vi "DAQ_Initialize.vi"(8 "error in":errorcluster, 11 "ai0 = Temperature\nai1 = Current\nai2 = Torque\nai3 = Vibration\nai4 = RPM":tag) -> (0 "error out":errorcluster, 3 "task out":refnum<k21>)   [LabVIEW 2026]
uses:
  <vilib>/DAQmx/create/channels.llb/DAQmx Create Channel (AI-Voltage-Basic).vi
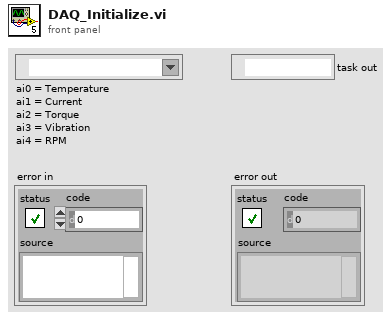
[diagram p1: front panel]
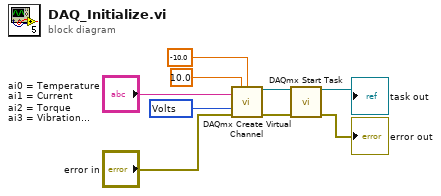
[diagram p0: block diagram]
diagram:
  w7 = 10348 items=["Volts"=10348, "From Custom Scale"=10065] ("units")
  n1 = call-poly <vilib>:"DAQmx Create Virtual Channel.vi"("maximum value"=10.0, "minimum value"=-10.0, "physical channels"="ai0 = Temperature\nai1 = Current\nai2 = Torque\nai3 = Vibration\nai4 = RPM", "units"=w7, "error in"="error in") -> ("task out"=w3:refnum<k21>, "error out"=w2:errorcluster)  [unwired: 9 in]
  n2 = call <vilib>:"DAQmx Start Task.vi"("task/channels in"=w3, "error in"=w2) -> ("task out"=→"task out":refnum<k21>, "error out"=→"error out":errorcluster)  [unwired: 12 in]
